vi "read_in_port.vi"() -> ()   [LabVIEW 2012]
doc: "Use this template to parse data acquired from an instrument attached to your computer through a GPIB, serial, or other port and write the data to a file. Note: VIs created from this template will have automatic error handling enabled by default."
uses:
  Usb_Daq_V52_Dll.dll
panel:
  in  "停止":bool
  out "led8":bool
  out "led7":bool
  out "led6":bool
  out "led5":bool
  out "led4":bool
  out "led3":bool
  out "led2":bool
  out "led1":bool
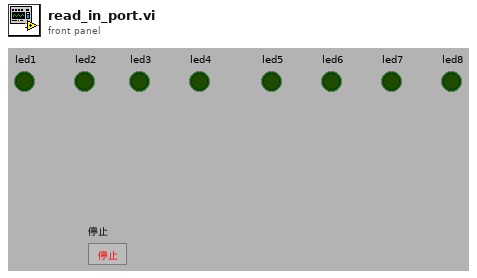
[diagram p1: front panel]
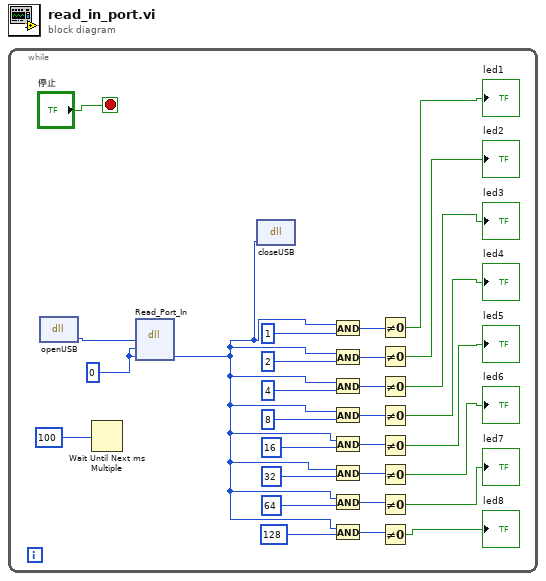
[diagram p0: block diagram]
diagram:
  n1 = while {
    stop <- "停止" stop-if-true
    w1 = u16 0
    n2 = dll-call lib="PTH1labs Ebackup数据采集卡uSB!USB数据采集卡资料HKUSB6203例程labviewUsb_Daq_V52_Dll.dll" fn="openUSB"() -> ("返回类型"=w4:i32)  [unwired: 3 in, 2 out]
    n3 = Wait Until Next ms Multiple(millisecond multiple=100) -> ()  [unwired: 1 out]
    n4 = dll-call lib="PTH1labs Ebackup数据采集卡uSB!USB数据采集卡资料HKUSB6203例程labviewUsb_Daq_V52_Dll.dll" fn="Read_Port_In"("返回类型"=w4, "dev"=w1, "in_port"=w1) -> ("in_port"=w3:u16)  [unwired: 4 in, 2 out]
    n5 = dll-call lib="PTH1labs Ebackup数据采集卡uSB!USB数据采集卡资料HKUSB6203例程labviewUsb_Daq_V52_Dll.dll" fn="closeUSB"("返回类型"=w3) -> ()  [unwired: 2 in, 3 out]
    n6 = And(x=w3, y=1) -> (x .and. y?=w20:i32)
    n7 = And(x=w3, y=2) -> (x .and. y?=w19:i32)
    n8 = And(x=w3, y=4) -> (x .and. y?=w18:i32)
    n9 = And(x=w3, y=8) -> (x .and. y?=w17:i32)
    n10 = And(x=w3, y=16) -> (x .and. y?=w16:i32)
    n11 = And(x=w3, y=32) -> (x .and. y?=w15:i32)
    n12 = And(x=w3, y=64) -> (x .and. y?=w14:i32)
    n13 = And(x=w3, y=128) -> (x .and. y?=w13:i32)
    n14 = Not Equal To 0?(x=w20) -> (x != 0?=→"led1":bool)
    n15 = Not Equal To 0?(x=w19) -> (x != 0?=→"led2":bool)
    n16 = Not Equal To 0?(x=w18) -> (x != 0?=→"led3":bool)
    n17 = Not Equal To 0?(x=w17) -> (x != 0?=→"led4":bool)
    n18 = Not Equal To 0?(x=w16) -> (x != 0?=→"led5":bool)
    n19 = Not Equal To 0?(x=w15) -> (x != 0?=→"led6":bool)
    n20 = Not Equal To 0?(x=w14) -> (x != 0?=→"led7":bool)
    n21 = Not Equal To 0?(x=w13) -> (x != 0?=→"led8":bool)
  }
